vi "MCListbox - Move Combo Box.vi"(9 "CellPosition":T1, 10 "Combo Box in":refnum<vi>, 11 "MulticolumnListbox in":refnum<vi>) -> (2 "Combo Box out":refnum<vi>, 3 "MulticolumnListbox out":refnum<vi>)   [LabVIEW 2013]
uses:
  <vilib>/Utility/miscctls.llb/LVRowAndColumnTypeDef.ctl
  <vilib>/Utility/miscctls.llb/LVSelectionTypeDef.ctl
panel:
  out "Selection Color":u32
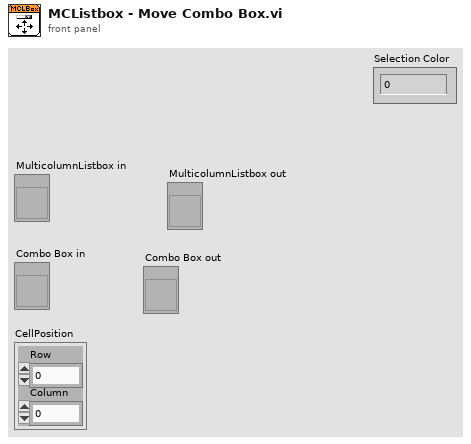
[diagram p1: front panel]
types:
  T1 = typedef "LVRowAndColumnTypeDef.ctl" = cluster{"Row":i32, "Column":i32}
  T2 = typedef "LVSelectionTypeDef.ctl" = cluster{"Selection Start":u32, "Selection End":u32}
  T3 = typedef "LVPositionTypeDef.ctl" = cluster{"Left":i32, "Top":i32}
  T4 = typedef "LVBoundsTypeDef.ctl" = cluster{"Width":u32, "Height":u32}
  T5 = typedef "LVRectTypeDef.ctl" = cluster{"Left":i16, "Top":i16, "Right":i16, "Bottom":i16}
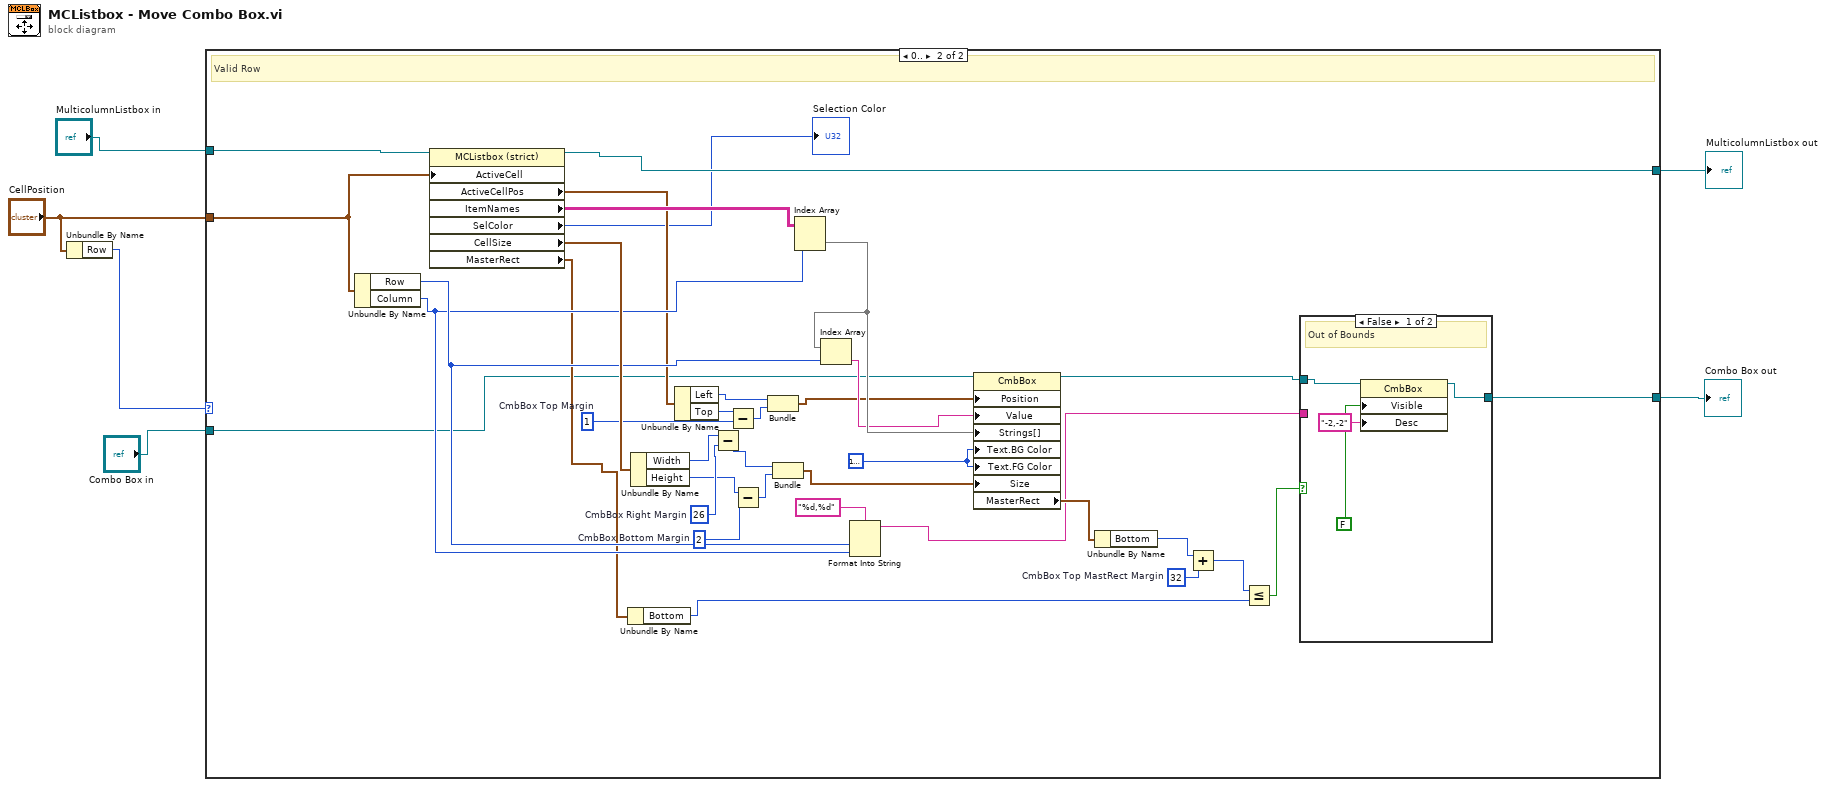
[diagram p0: block diagram]
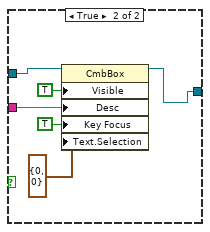
[diagram p3: hidden frame]
diagram:
  n1 = Unbundle By Name("CellPosition") -> ("Row"=w5:i32)
  n2 = case shown="0.." w5 {
    tunnel: "CellPosition" -> [_ w15]
    tunnel: "Combo Box in" -> [w7 w14]
    tunnel: "MulticolumnListbox in" -> [w8 w13]
    tunnel: [w8 w12] -> w2
    tunnel: [w7 w11] -> w1
    frame -1, Default {
    }
    frame 0.. {
      w10 = u32 16777216 ("Color Box")
      w21 = u32 32  # CmbBox Top MastRect Margin
      w27 = 1  # CmbBox Top Margin
      w33 = u32 2  # CmbBox Bottom Margin
      w39 = u32 26  # CmbBox Right Margin
      # "Valid Row"
      n3 = Unbundle By Name(w15) -> ("Row"=w35:i32, "Column"=w34:i32)
      n4 = property class="MCListbox (strict)"(reference=w13, "ActiveCell"=w15) -> (reference out=w12:refnum<vi>, "ActiveCellPos"=w31:T3, "ItemNames"=w37:string[][], "SelColor"=→"Selection Color":u32, "CellSize"=w38:T4, "MasterRect"=w24:T5)  [unwired: 1 in, 1 out]
      n5 = Unbundle By Name(w24) -> ("Bottom"=w19:i16)
      n6 = Unbundle By Name(w38) -> ("Width"=w41:u32, "Height"=w25:u32)
      n7 = Unbundle By Name(w31) -> ("Left"=w29:i32, "Top"=w28:i32)
      n8 = Subtract(x=w41, y=w39) -> (x-y=w42:u32)
      n9 = Subtract(x=w28, y=w27) -> (x-y=w26:i32)
      n10 = Subtract(x=w25, y=w33) -> (x-y=w32:u32)
      n11 = Bundle("Left"=w29, w26) -> (w30:cluster{"Left":i32, i32})  [unwired: 1 in]
      n12 = Bundle(w42, w32) -> (w40:cluster{u32, u32})  [unwired: 1 in]
      n13 = Index Array(array=w37, index (col)=w34) -> (element=w44:string[])  [unwired: 1 in]
      n14 = Index Array(array=w44, index=w35) -> (element=w43:string)
      n15 = Format Into String(format string="%d,%d", w35, w34) -> (resulting string=w16:string)  [unwired: 2 in, 1 out]
      n16 = property on="Property Node" class="CmbBox"(reference=w14, "Position"=w30, "Value"=w43, "Strings[]"=w44, "Text.BG Color"=w10, "Text.FG Color"=w10, "Size"=w40) -> (reference out=w17:refnum<vi>, "MasterRect"=w23:T5)  [unwired: 1 in, 1 out]
      n17 = Unbundle By Name(w23) -> ("Bottom"=w22:i16)
      n18 = Add(x=w22, y=w21) -> (x+y=w20:u32)
      n19 = Less Or Equal?(x=w20, y=w19) -> (x <= y?=w18:bool)
      n20 = case shown="False" w18 {
        tunnel: w17 -> [w47 w54]
        tunnel: [w46 w53] -> w11
        tunnel: w16 -> [_ w51]
        frame False {
          # "Out of Bounds"
          n21 = property on="Property Node" class="CmbBox"(reference=w47, "Visible"=FALSE, "Desc"="-2,-2" ("Description")) -> (reference out=w46:refnum<vi>)  [unwired: 1 in, 1 out]
        }
        frame True {
          n22 = property on="Property Node" class="CmbBox"(reference=w54, "Visible"=TRUE, "Desc"=w51, "Key Focus"=TRUE, "Text.Selection"=T2 {"Selection Start"=0, "Selection End"=0}) -> (reference out=w53:refnum<vi>)  [unwired: 1 in, 1 out]
        }
      }
    }
  }
  "MulticolumnListbox out" <- w2
  "Combo Box out" <- w1
